vi "conditioning_behavior_3s_post_stim.vi"() -> ()   [LabVIEW 2019]
doc: "The myRIO Project template acquires acceleration data from the onboard accelerometer and displays the changes of acceleration values in a waveform chart."
uses:
  <vilib>/Analysis/Matrix/Datatypes/RealMatrix.ctl
  <vilib>/myRIO/Common/Instrument Driver Framework/myRIO v1.0/Encoder/typedefs/Encoder Signal Mode.ctl
  <vilib>/myRIO/Instrument Drivers/Onboard IO/Encoder/typedefs/Encoder Reference.ctl
  <vilib>/myRIO/Common/Instrument Driver Framework/Utilities/typedefs/myRIO Generic Hardware Reference.ctl
  <vilib>/myRIO/Common/Instrument Driver Framework/Utilities/typedefs/Hardware Version Enum.ctl
  <vilib>/myRIO/Common/Instrument Driver Framework/Utilities/typedefs/myRIO v1.0 Reference.ctl
  <vilib>/myRIO/Common/Instrument Driver Framework/Utilities/typedefs/Generic FPGA Reference.ctl
  <vilib>/myRIO/Common/Instrument Driver Framework/myRIO v1.0/Encoder/typedefs/Encoder Channels Enum.ctl
  <vilib>/myRIO/Common/Instrument Driver Framework/myRIO v1.0/Encoder/typedefs/Encoder Configuration v1.0.ctl
  <vilib>/userdefined/High Color/nirio_resource_hc.ctl
  <vilib>/myRIO/Instrument Drivers/Onboard IO/DIO/typedefs/DIO Reference.ctl
  <vilib>/myRIO/Common/Instrument Driver Framework/myRIO v1.0/DIO/typedefs/DIO Channels List.ctl
  <vilib>/myRIO/Common/Instrument Driver Framework/myRIO v1.0/DIO/typedefs/DIO Channels Enum.ctl
  <vilib>/myRIO/Common/Instrument Driver Framework/Utilities/vis/Is FPGA Ref Available.vi
  <vilib>/myRIO/Common/Instrument Driver Framework/myRIO v1.0/Encoder/vis/myRIO v1.1 Open Encoder.vi
  <vilib>/myRIO/Instrument Drivers/Onboard IO/Encoder/vis/Read.vi
  <vilib>/myRIO/Common/Instrument Driver Framework/myRIO v1.0/DIO/vis/myRIO v1.1 Open DIO.vi
  <vilib>/myRIO/Instrument Drivers/Onboard IO/DIO/vis/Write.vi
  <vilib>/myRIO/Instrument Drivers/Onboard IO/DIO/vis/Read.vi
  <vilib>/myRIO/Common/Instrument Driver Framework/Utilities/vis/Validate Channels.vi
  <vilib>/myRIO/Common/Instrument Driver Framework/myRIO v1.0/Encoder/vis/myRIO v1.0 Reserve Encoder.vi
  <vilib>/myRIO/Common/Instrument Driver Framework/myRIO v1.0/DIO/vis/myRIO v1.0 Reserve DIO.vi
  <vilib>/myRIO/Common/Instrument Driver Framework/myRIO v1.0/Encoder/vis/myRIO v1.0 Build MUX Configuration Encoder.vi
  <vilib>/myRIO/Common/Instrument Driver Framework/myRIO v1.0/Resource Manager/vis/myRIO v1.0 Reserve Channel List.vi
  <vilib>/myRIO/Common/Instrument Driver Framework/myRIO v1.0/DIO/vis/myRIO v1.0 Build MUX Configuration DIO.vi
  <vilib>/myRIO/Common/Instrument Driver Framework/myRIO v1.0/Resource Manager/vis/myRIO v1.0 Create Configuration List.vi
  <vilib>/myRIO/Common/Instrument Driver Framework/myRIO v1.0/Resource Manager/vis/myRIO v1.0 Reserve Channel.vi
  <vilib>/myRIO/Common/Instrument Driver Framework/myRIO v1.0/Resource Manager/vis/myRIO v1.0 Unreserve Channel.vi
  <vilib>/myRIO/Common/Instrument Driver Framework/myRIO v1.0/Resource Manager/vis/myRIO v1.0 Build Mutex Name.vi
  <vilib>/Utility/VariantDataType/GetNumericInfo.vi
  <vilib>/Utility/error.llb/Error Cluster From Error Code.vi
  <vilib>/myRIO/Common/Instrument Driver Framework/myRIO v1.0/myRIO v1.1 Open.vi
  <vilib>/myRIO/Common/Instrument Driver Framework/Utilities/vis/IO Manager.vi
  <vilib>/myRIO/Common/Instrument Driver Framework/Utilities/vis/Configuration Manager.vi
  <vilib>/myRIO/Common/Instrument Driver Framework/myRIO v1.0/Resource Manager/vis/myRIO v1.0 Configure IO.vi
  <vilib>/myRIO/Common/Instrument Driver Framework/myRIO v1.0/myRIO v1.0 Close.vi
  <vilib>/myRIO/Common/Instrument Driver Framework/myRIO v1.0/Encoder/vis/myRIO v1.0 Configure Encoder.vi
  <vilib>/myRIO/Common/Instrument Driver Framework/myRIO v1.0/Encoder/vis/myRIO v1.0 Read Encoder.vi
  <vilib>/myRIO/Common/Instrument Driver Framework/myRIO v1.0/DIO/vis/myRIO v1.0 Read DIO.vi
  <vilib>/myRIO/Common/Instrument Driver Framework/myRIO v1.0/DIO/vis/myRIO v1.0 Write DIO.vi
  <vilib>/myRIO/Express VI/Onboard IO/Encoder/Encoder Express VI.xnode
  <vilib>/myRIO/Instrument Drivers/Onboard IO/Encoder/vis/myRIO Encoder Open.xnode
  <vilib>/myRIO/Express VI/Onboard IO/DI/DI Express VI.xnode
  <vilib>/myRIO/Instrument Drivers/Onboard IO/DIO/vis/myRIO DIO Open.xnode
  <vilib>/myRIO/Express VI/Onboard IO/DO/DO Express VI.xnode
  <vilib>/myRIO/Instrument Drivers/Onboard IO/Encoder/Encoder.lvlib
  <vilib>/myRIO/Instrument Drivers/Onboard IO/DIO/DIO.lvlib
  <vilib>/Analysis/Matrix/NI_Matrix.lvlib
panel:
  out "Array temp2":T1
  out "Stimuli Loaded":bool
  out "Stim_ID":dbl[](array[numeric])
  out "Reward_mat":dbl[](array[numeric])
  out "Reward":bool=TRUE
  out "Frame clock":i32
  out "Licks":u32
  out "Lick":bool
  out "Time":dbl
  out "Stop":bool
  in  "Frames to collect":u32
  out "Overflow?":bool
  out "Counter Value":i32
  out "Velocity":dbl
  out "Velocity Plot":dbl[](graph)
  out "Velocity array":dbl[](array[numeric])
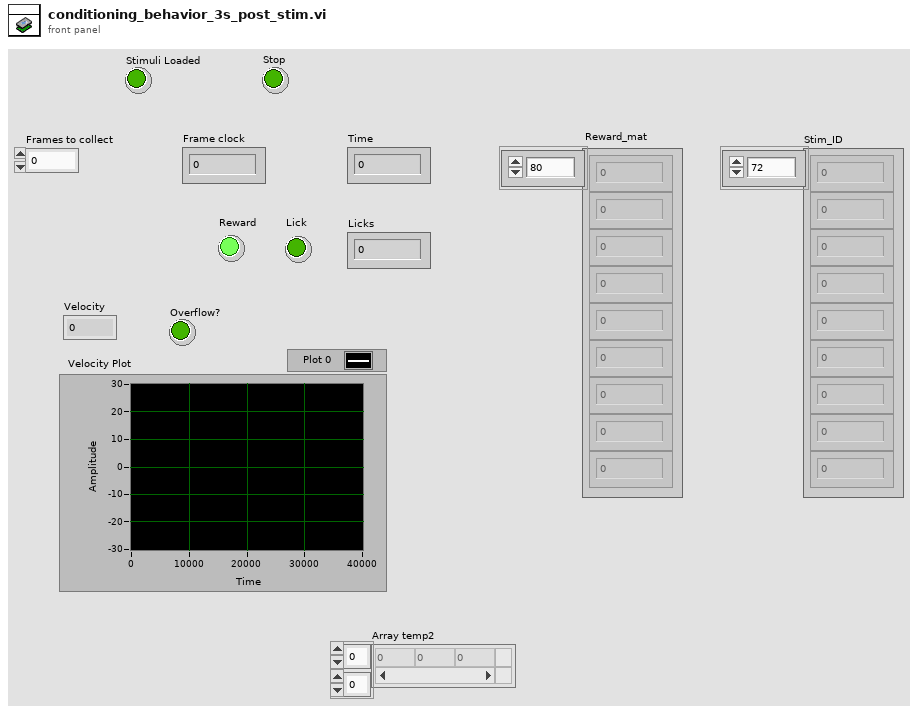
[diagram p1: front panel]
types:
  T1 = typedef "NI_Matrix.lvlib/RealMatrix.ctl" = dbl[][]
  T2 = typedef "Encoder.lvlib/Encoder Reference.ctl" = cluster{"myRIO Reference":T3, "Encoder Channels Enum":T7}
  T3 = typedef "myRIO Generic Hardware Reference.ctl" = cluster{"myRIO Model":T4, "myRIO Hardware Reference":T5}
  T4 = typedef "Hardware Version Enum.ctl" = enum16{"Unknown", "myRIO-1900", "myRIO-1950", "roboRIO", "NI ELVIS RIO CM", "ELVIS III"}
  T5 = typedef "myRIO v1.0 Reference.ctl" = cluster{"Generic FPGA Reference":T6, "Allow multiple opens":bool}
  T6 = typedef "Generic FPGA Reference.ctl" = refnum<k20>
  T7 = typedef "Encoder Channels Enum.ctl" = enum16{"Not Connected", "C/ENC0", "C/ENC1", "A/ENC", "A/ENC0", "A/ENC1", "A/ENC2", "A/ENC3", "A/ENC4", "A/ENC5", "A/ENC6", "A/ENC7", "A/ENC8", "A/ENC9", "B/ENC", "B/ENC0", "B/ENC1", "B/ENC2", "B/ENC3", "B/ENC4", "B/ENC5", "B/ENC6", "B/ENC7", "B/ENC8", "B/ENC9", "DIO/ENC0", "DIO/ENC1", "DIO/ENC2", "DIO/ENC3", "DIO/ENC4"}
  T8 = typedef "Encoder Signal Mode.ctl" = enum16{"Quadrature phase signal", "Step and direction signal"}
  T9 = typedef "nirio_resource_hc.ctl" = tag
  T10 = typedef "DIO.lvlib/DIO Reference.ctl" = cluster{"myRIO Reference":T3, "DIO Channels List":T11}
  T11 = typedef "DIO Channels List.ctl" = T12[]
  T12 = typedef "DIO Channels Enum.ctl" = enum16{"Not Connected", "C/DIO0", "C/DIO1", "C/DIO2", "C/DIO3", "C/DIO4", "C/DIO5", "C/DIO6", "C/DIO7", "A/DIO0", "A/DIO1", "A/DIO2", "A/DIO3", "A/DIO4", "A/DIO5", "A/DIO6", "A/DIO7", "A/DIO8", "A/DIO9", "A/DIO10", "A/DIO11", "A/DIO12", "A/DIO13", "A/DIO14", "A/DIO15", "A/DIO16", "A/DIO17", "A/DIO18", "A/DIO19", "B/DIO0", "B/DIO1", "B/DIO2", "B/DIO3", "B/DIO4", "B/DIO5", "B/DIO6", "B/DIO7", "B/DIO8", "B/DIO9", "B/DIO10", "B/DIO11", "B/DIO12", "B/DIO13", "B/DIO14", "B/DIO15", "B/DIO16", "B/DIO17", "B/DIO18", "B/DIO19", "LED0", "LED1", "LED2", "LED3", "Button0", "DIO/DIO0", "DIO/DIO1", "DIO/DIO2", "DIO/DIO3", "DIO/DIO4", "DIO/DIO5", "DIO/DIO6", "DIO/DIO7", "DIO/DIO8", "DIO/DIO9", "SPI/CS0", "SPI/CS1", "SPI/CS2", "SPI/CS3", "LED RADIO (Green)", "LED RADIO (Red)", "LED COMM (Green)", "LED COMM (Red)", "LED MODE (Green)", "LED MODE (Red)"}
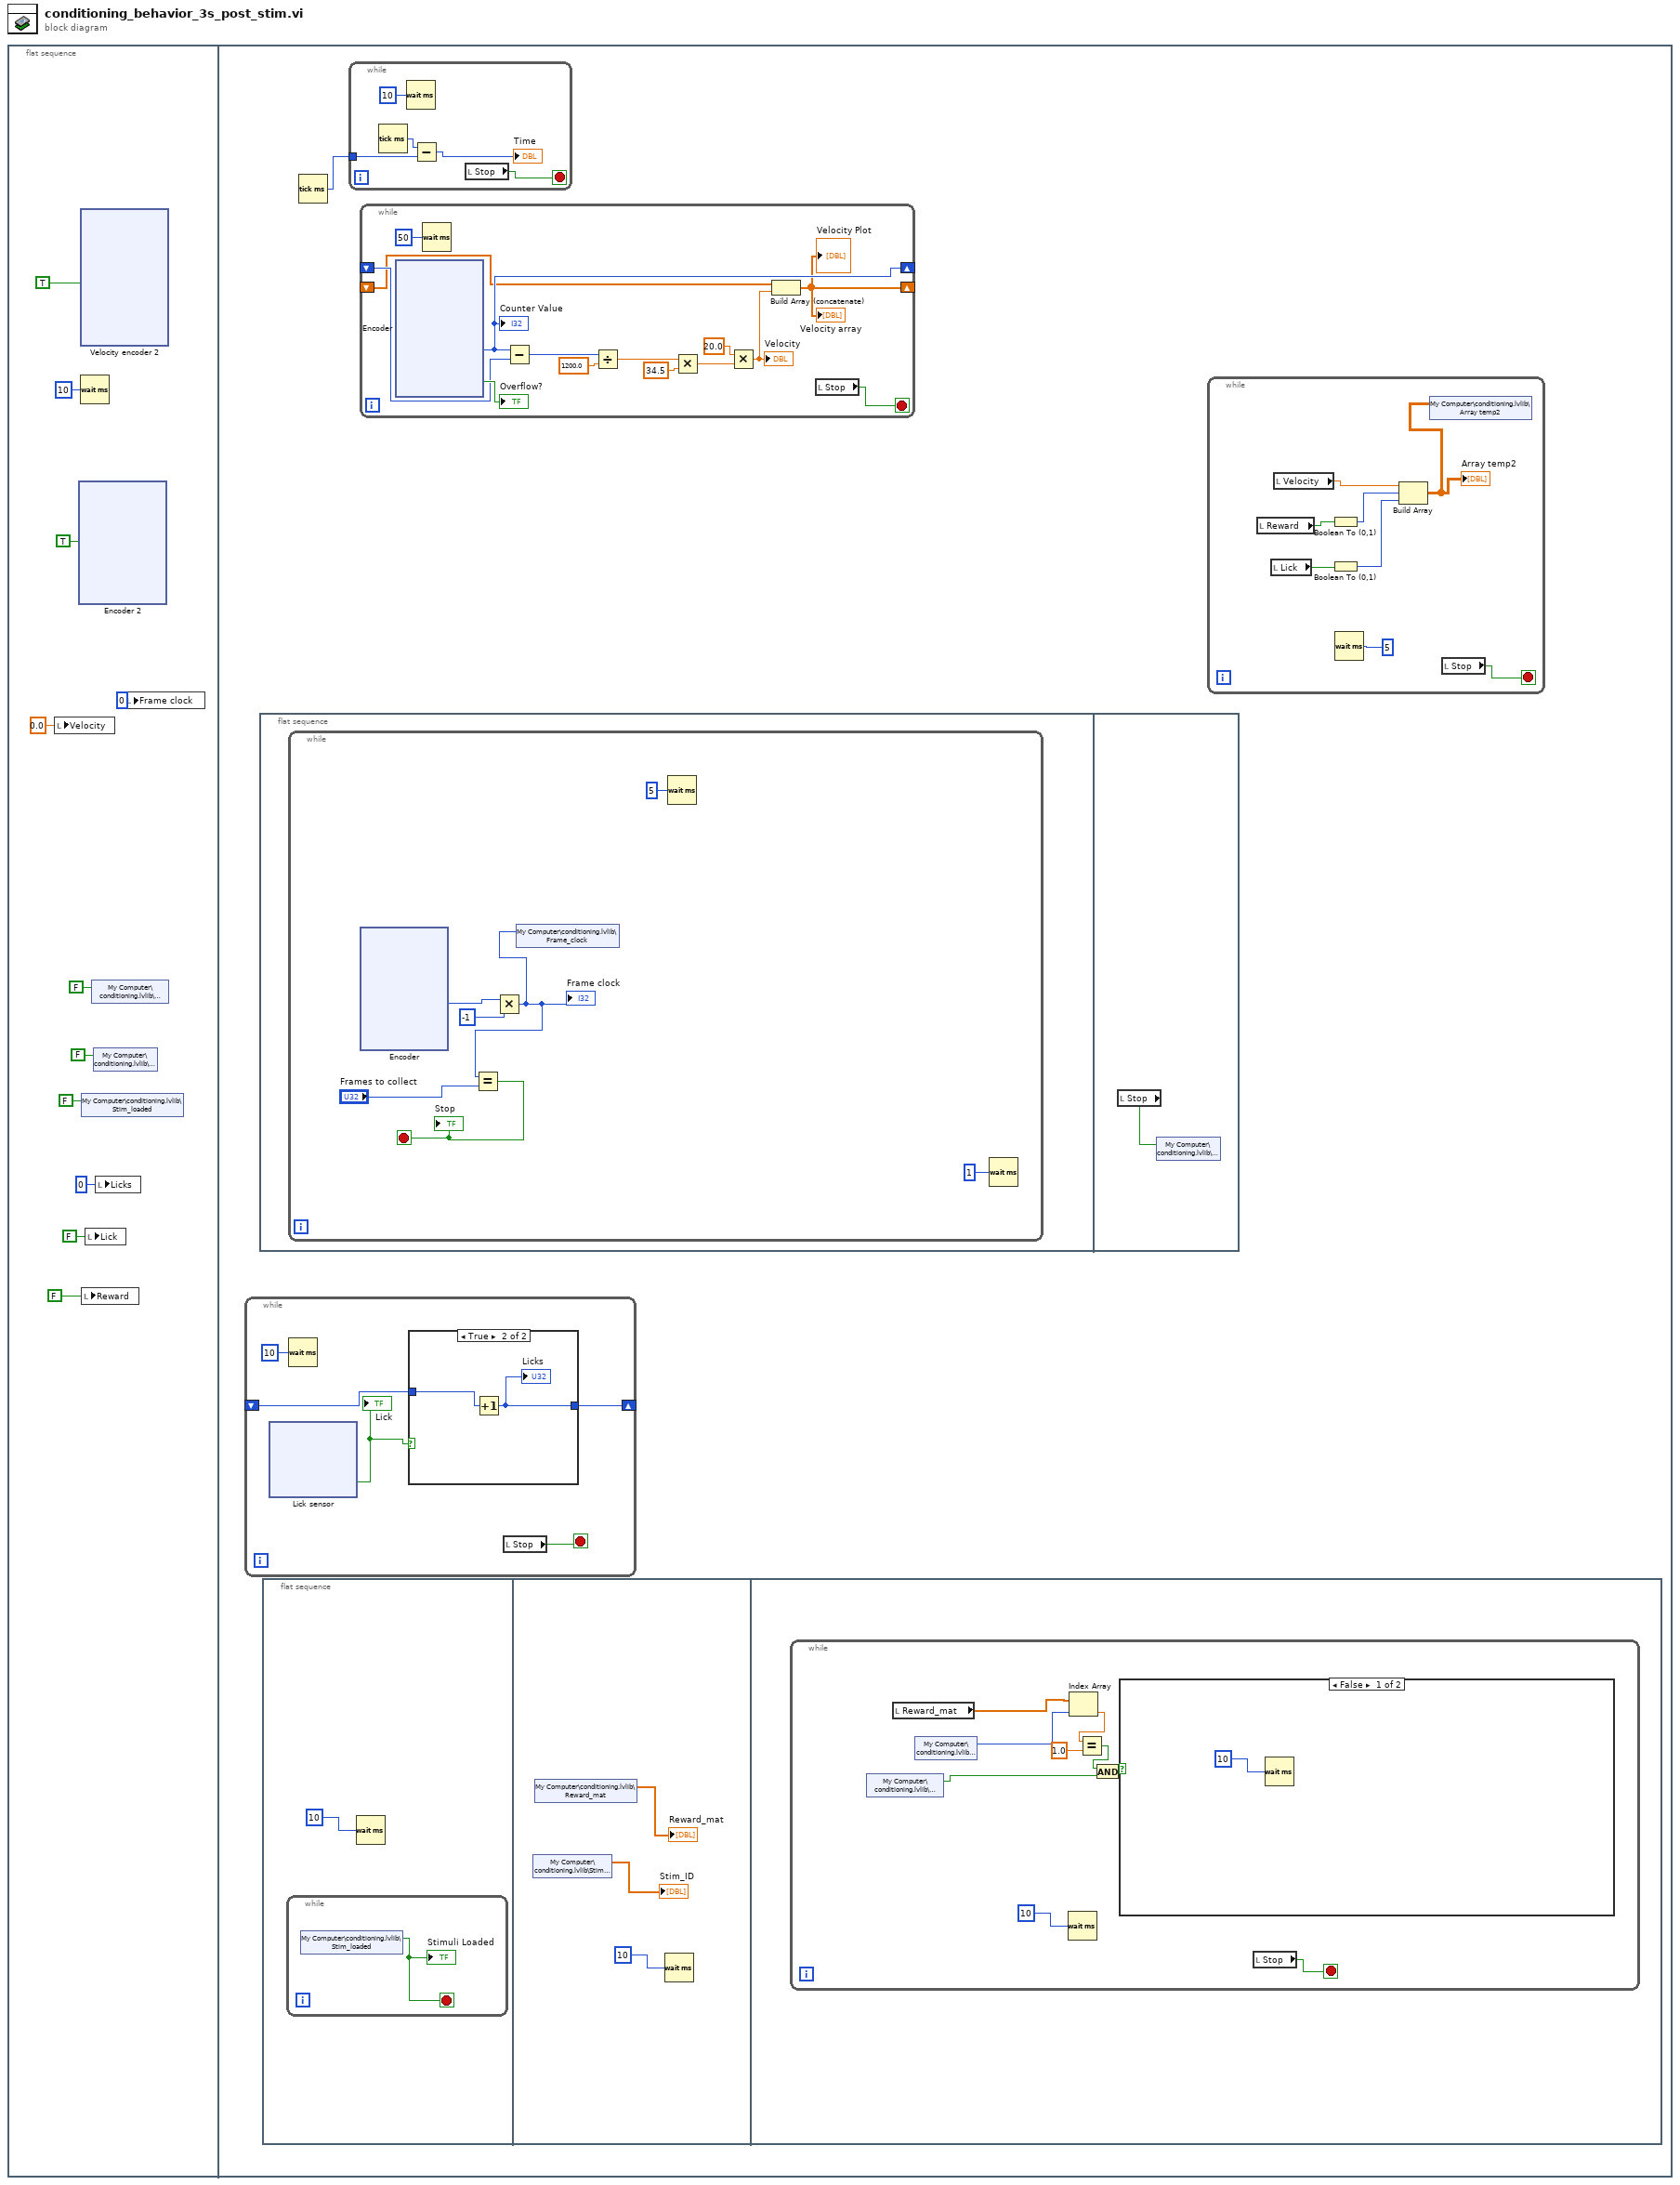
[diagram p0: block diagram]
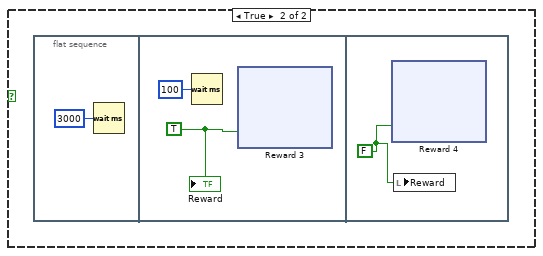
[diagram p2: hidden frame]
diagram:
  n1 = flat-sequence {
    frame #0 {
      n2 = local write "Velocity"(0.0 ("Velocity")) -> ()
      n3 = xnode "Encoder 2"("Reset Counter"=TRUE) -> ()  [unwired: 1 in, 4 out]
      n4 = xnode "Velocity encoder 2"("Reset Counter"=TRUE) -> ()  [unwired: 1 in, 4 out]
      n5 = Wait (ms)(milliseconds to wait=u32 10) -> ()  [unwired: 1 out]
      n6 = shared-variable "My Computer\\conditioning.lvlib\\Stim_loaded"(FALSE ("Stim_loaded")) -> ()  [unwired: 1 in, 1 out]
      n7 = local write "Reward"(FALSE ("Give reward")) -> ()
      n8 = local write "Lick"(FALSE ("Lick")) -> ()
      n9 = shared-variable "My Computer\\conditioning.lvlib\\Display"(FALSE ("Display")) -> ()  [unwired: 1 in, 1 out]
      n10 = shared-variable "My Computer\\conditioning.lvlib\\Stop"(FALSE ("Stop")) -> ()  [unwired: 1 in, 1 out]
      n11 = local write "Licks"(u32 0 ("Licks")) -> ()
      n12 = local write "Frame clock"(u32 0 ("Frames")) -> ()
    }
    frame #1 {
      n13 = while {
        shift-right: [w258] -> _
        shift-left: _ -> [w257]
        stop <- w256 stop-if-true
        n14 = xnode "Lick sensor"() -> ("C/DIO1 (DIO1)"=w259:bool)  [unwired: 1 in, 1 out]
        "Lick" <- w259
        n15 = Wait (ms)(milliseconds to wait=u32 10) -> ()  [unwired: 1 out]
        n16 = case shown="True" w259 {
          tunnel: [w261 w263] -> w258
          tunnel: w257 -> [w261 w262]
          frame False {
          }
          frame True {
            n17 = Increment(x=w262) -> (x+1=w263:u32)
            "Licks" <- w263
          }
        }
        n18 = local read "Stop"() -> (w256:bool)
      }
      n19 = flat-sequence {
        frame #0 {
          n20 = while {
            stop <- w203 stop-if-true
            n21 = xnode "Encoder"() -> ("Counter Value"=w207:i32)  [unwired: 2 in, 3 out]
            n22 = Multiply(x=w207, y=-1) -> (x*y=w202:i32)
            "Frame clock" <- w202
            n23 = Equal?(x=w202, y="Frames to collect") -> (x = y?=w203:bool)
            "Stop" <- w203
            n24 = shared-variable "My Computer\\conditioning.lvlib\\Frame_clock"(w202) -> ()  [unwired: 1 in, 1 out]
            n25 = Wait (ms)(milliseconds to wait=u32 5) -> ()  [unwired: 1 out]
            n26 = Wait (ms)(milliseconds to wait=u32 1) -> ()  [unwired: 1 out]
          }
        }
        frame #1 {
          n27 = local read "Stop"() -> (w255:bool)
          n28 = shared-variable "My Computer\\conditioning.lvlib\\Stop"(w255) -> ()  [unwired: 1 in, 1 out]
        }
      }
      n29 = flat-sequence {
        frame #0 {
          n30 = while {
            stop <- w114 stop-if-true
            n31 = shared-variable "My Computer\\conditioning.lvlib\\Stim_loaded"() -> (w114:bool)  [unwired: 1 in, 1 out]
            "Stimuli Loaded" <- w114
          }
          n32 = Wait (ms)(milliseconds to wait=u32 10) -> ()  [unwired: 1 out]
        }
        frame #1 {
          n33 = shared-variable "My Computer\\conditioning.lvlib\\Stim_ID"() -> (→"Stim_ID":dbl[])  [unwired: 1 in, 1 out]
          n34 = shared-variable "My Computer\\conditioning.lvlib\\Reward_mat"() -> (→"Reward_mat":dbl[])  [unwired: 1 in, 1 out]
          n35 = Wait (ms)(milliseconds to wait=u32 10) -> ()  [unwired: 1 out]
        }
        frame #2 {
          n36 = while {
            stop <- w122 stop-if-true
            n37 = shared-variable "My Computer\\conditioning.lvlib\\Display"() -> (w118:bool)  [unwired: 1 in, 1 out]
            n38 = local read "Reward_mat"() -> (w121:dbl[])
            n39 = shared-variable "My Computer\\conditioning.lvlib\\Trial"() -> (w119:u32)  [unwired: 1 in, 1 out]
            n40 = Wait (ms)(milliseconds to wait=u32 10) -> ()  [unwired: 1 out]
            n41 = Index Array(array=w121, index=w119) -> (element=w120:dbl)
            n42 = Equal?(x=w120, y=1.0) -> (x = y?=w124:bool)
            n43 = And(x=w124, y=w118) -> (x .and. y?=w123:bool)
            n44 = case shown="False" w123 {
              frame False {
                n45 = Wait (ms)(milliseconds to wait=u32 10) -> ()  [unwired: 1 out]
              }
              frame True {
                n46 = flat-sequence {
                  frame #0 {
                    n47 = Wait (ms)(milliseconds to wait=u32 3000) -> ()  [unwired: 1 out]
                  }
                  frame #1 {
                    w129 = TRUE ("C/DIO0 (DIO0)")
                    n48 = Wait (ms)(milliseconds to wait=u32 100) -> ()  [unwired: 1 out]
                    n49 = xnode "Reward 3"("C/DIO0 (DIO0)"=w129) -> ()  [unwired: 1 in, 1 out]
                    "Reward" <- w129
                  }
                  frame #2 {
                    w166 = FALSE ("C/DIO0 (DIO0)")
                    n50 = xnode "Reward 4"("C/DIO0 (DIO0)"=w166) -> ()  [unwired: 1 in, 1 out]
                    n51 = local write "Reward"(w166) -> ()
                  }
                }
              }
            }
            n52 = local read "Stop"() -> (w122:bool)
          }
        }
      }
      n53 = Tick Count (ms)() -> (millisecond timer value=w104:u32)
      n54 = while {
        tunnel: w104 -> [w362]
        stop <- w359 stop-if-true
        n55 = Tick Count (ms)() -> (millisecond timer value=w363:u32)
        n56 = Wait (ms)(milliseconds to wait=u32 10) -> ()  [unwired: 1 out]
        n57 = Subtract(x=w363, y=w362) -> (x-y=→"Time":u32)
        n58 = local read "Stop"() -> (w359:bool)
      }
      n59 = while {
        shift-right: [w309] -> _
        shift-left: _ -> [w310]
        shift-right: [w301] -> _
        shift-left: _ -> [w300]
        stop <- w299 stop-if-true
        n60 = xnode "Encoder"() -> ("Counter Value"=w309:i32, "Overflow?"=→"Overflow?":bool)  [unwired: 2 in, 2 out]
        "Counter Value" <- w309
        n61 = Wait (ms)(milliseconds to wait=u32 50) -> ()  [unwired: 1 out]
        n62 = Subtract(x=w309, y=w310) -> (x-y=w302:i32)
        n63 = Divide(x=w302, y=1200.0 ("600")) -> (x/y=w307:dbl)
        n64 = Multiply(x=w307, y=34.5) -> (x*y=w305:dbl)
        n65 = Multiply(x=20.0, y=w305) -> (x*y=w303:dbl)
        "Velocity" <- w303
        n66 = Build Array (concatenate)(w300, w303) -> (w301:dbl[])
        "Velocity Plot" <- w301
        "Velocity array" <- w301
        n67 = local read "Stop"() -> (w299:bool)
      }
      n68 = while {
        stop <- w106 stop-if-true
        n69 = local read "Reward"() -> (w111:bool)
        n70 = local read "Lick"() -> (w112:bool)
        n71 = local read "Velocity"() -> (w110:dbl)
        n72 = Boolean To (0,1)(Boolean=w111) -> (0, 1=w109:i16)
        n73 = Boolean To (0,1)(Boolean=w112) -> (0, 1=w108:i16)
        n74 = Wait (ms)(milliseconds to wait=u32 5) -> ()  [unwired: 1 out]
        n75 = Build Array(w110, w109, w108) -> (w105:T1)
        "Array temp2" <- w105
        n76 = shared-variable "My Computer\\conditioning.lvlib\\Array temp2"(w105) -> ()  [unwired: 1 in, 1 out]
        n77 = local read "Stop"() -> (w106:bool)
      }
    }
  }
